vi "MTM2_getSample_powerStatus.vi"(8 "error in (no error)":errorcluster, 11 "powerStatus_Ctl":T1) -> (0 "error out":errorcluster, 2 "function return":i32, 3 "powerStatus_Ctl out":T1)   [LabVIEW 2018, in "SALLV_MTM2.lvlib"]
doc: "int MTM2_shm_getSample_powerStatusLV(MTM2_powerStatusLV *powerStatus_Ctl );"
uses:
  DataTypes/powerStatus.ctl
  SALLV_MTM2.lvlib
  SALLV_MTM2.so
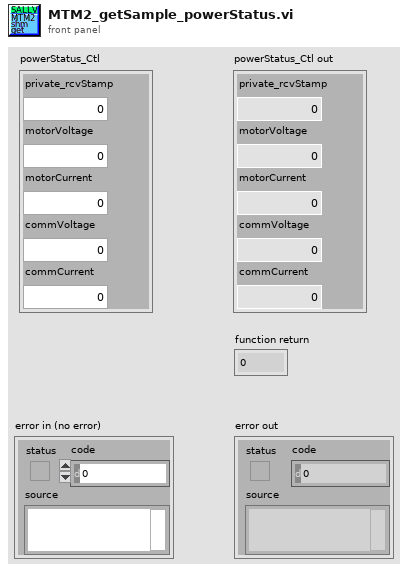
[diagram p1: front panel]
types:
  T1 = typedef "SALLV_MTM2.lvlib/powerStatus.ctl" = cluster{"private_rcvStamp":dbl, "motorVoltage":dbl, "motorCurrent":dbl, "commVoltage":dbl, "commCurrent":dbl}
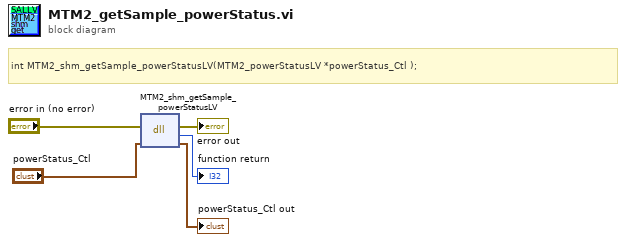
[diagram p0: block diagram]
diagram:
  # "int MTM2_shm_getSample_powerStatusLV(MTM2_powerStatusLV *powerStatus_Ctl );"
  n1 = dll-call lib="home/ttsai/Documents/salTestLabViewApi/SALLV_MTM2/SALLV_MTM2.*" fn="MTM2_shm_getSample_powerStatusLV"(error in="error in (no error)", "powerStatus_Ctl"="powerStatus_Ctl") -> (error out=→"error out":errorcluster, →"function return":i32, "powerStatus_Ctl"=→"powerStatus_Ctl out":T1)  [unwired: 2 in, 1 out]
